vi "Update Plot Name.vi"(8 "error in (no error)":errorcluster, 10 "NewVal":cluster{"String":string, "Picture":picture}[](array[cluster]), 11 "2D Plot.lvclass in":refnum<class "2D Plot.lvclass">) -> (0 "error out":errorcluster, 3 "2D Plot.lvclass out":refnum<class "2D Plot.lvclass">)   [LabVIEW 2017, in "2D Plot.lvclass"]
uses:
  <vilib>/Math Plots/2D Math Plots/2D Plot/2D Plot/2D Plot.lvclass
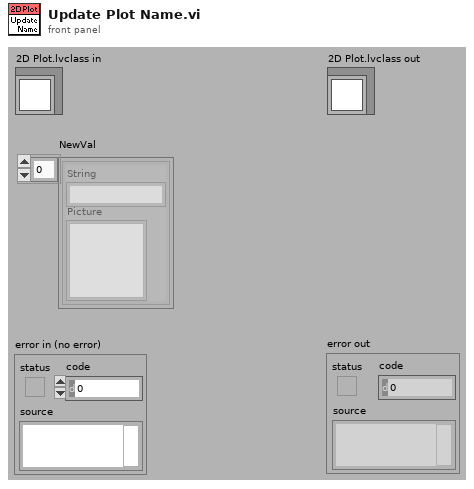
[diagram p1: front panel]
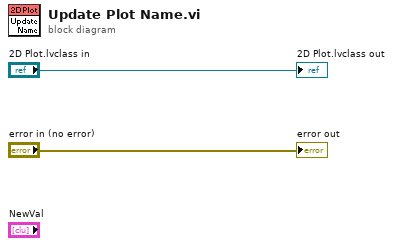
[diagram p0: block diagram]
diagram:
  "2D Plot.lvclass out" <- "2D Plot.lvclass in"
  "error out" <- "error in (no error)"
